vi "T.vi"(6 "Data Input(Hex)":string="000007d100000000", 8 "错误输入（无错误）":errorcluster, 9 "ID(Hex 高位有效)":string="00000182", 10 "CANChannel":u32) -> (0 "错误输出":errorcluster, 2 "Result":bool)   [LabVIEW 2013]
uses:
  InitConfig.ctl
  DevType.ctl
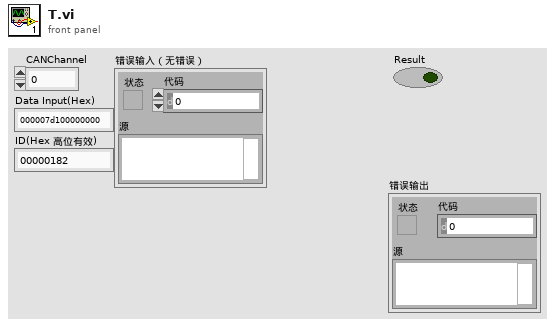
[diagram p1: front panel]
types:
  T1 = typedef "DevType.ctl" = u16
  T2 = typedef "InitConfig.ctl" = cluster{"AccCode":u32, "AccMask":u32, "Reserved":u32, "Filter":u8, "kCanBaud":u8, "Timing0":u8, "Timing1":u8, "Mode":u8, "CanRx_IER":u8}
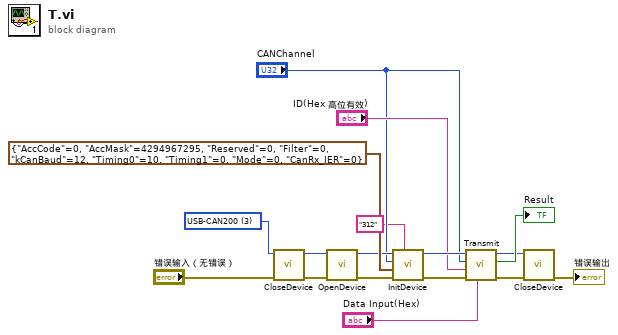
[diagram p0: block diagram]
diagram:
  w16 = T1 3 items=["PCI-CAN200"=7, "USB-CAN"=2, "USB-CAN200"=3] ("DeviceType")
  n1 = call "CloseDevice.vi"("错误输入（无错误）"="错误输入（无错误）", "DeviceType"=w16) -> ("错误输出"=w7:errorcluster, "DeviceTypeOut"=w15:u16)  [unwired: 7 in, 1 out]
  n2 = call "OpenDevice.vi"("错误输入（无错误）"=w7, "DeviceType"=w15) -> ("错误输出"=w8:errorcluster, "DeviceTypeOut"=w14:u16)  [unwired: 7 in, 1 out]
  n3 = call "InitDevice.vi"("ID(Hex 高位有效)"="312", "错误输入（无错误）"=w8, "InitConfig"=T2 {"AccCode"=0, "AccMask"=4294967295, "Reserved"=0, "Filter"=0, "kCanBaud"=12, "Timing0"=10, "Timing1"=0, "Mode"=0, "CanRx_IER"=0}, "CanChannel"="CANChannel", "DeviceType"=w14) -> ("错误输出"=w9:errorcluster, "DeviceTypeOut"=w13:u16)  [unwired: 4 in, 1 out]
  n4 = call "Transmit.vi"("Data Input(Hex)"="Data Input(Hex)", "错误输入（无错误）"=w9, "ID(Hex 高位有效)"="ID(Hex 高位有效)", "CANChannel"="CANChannel", "DeviceType"=w13) -> ("错误输出"=w2:errorcluster, "Result"=→"Result":bool, "DeviceTypeOut"=w6:u16)  [unwired: 4 in]
  n5 = call "CloseDevice.vi"("错误输入（无错误）"=w2, "DeviceType"=w6) -> ("错误输出"=→"错误输出":errorcluster)  [unwired: 7 in, 2 out]
